vi "GetControlValue_DBL.vi"(8 "error in (no error)":errorcluster, 9 "Expected Data Type":dbl, 10 "Control Label":string, 11 "CtlLookup In":T1) -> (0 "error out":errorcluster, 2 "Value":dbl, 3 "CtlLookup Out":T1)   [LabVIEW 2018, in "CtlReferences.lvlib" / "CtlReferences.lvclass"]
doc: "This VI uses the GetControlByReference to get the specified control as a DBL"
uses:
  CtlReferences.lvclass
  TypeDefs/CtlLookup.ctl
  CtlReferences.lvclass/CtlReferences.ctl
  GetControlRef/GetControl_Control.vi
  GetControlRef/GetCtlRef_Base.vi
  GetCtlRef_Lookup.vi
  <vilib>/Utility/error.llb/Error Cluster From Error Code.vi
  Error_ToSpecificClass.vi
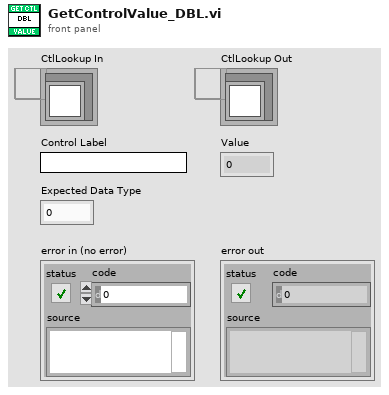
[diagram p1: front panel]
types:
  T1 = typedef "CtlReferences.lvlib/CtlReferences.lvclass/CtlLookup.ctl" = refnum<data-value>
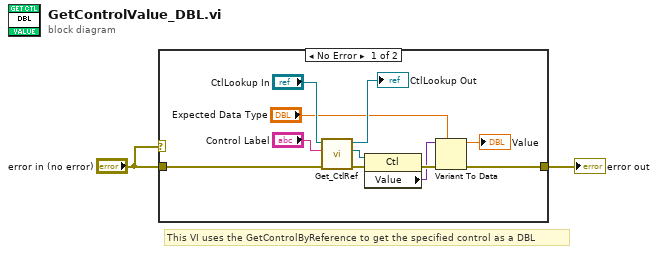
[diagram p0: block diagram]
diagram:
  # "This VI uses the GetControlByReference to get the specified control as a DBL"
  n1 = case shown="No Error" "error in (no error)" {
    tunnel: "error in (no error)" -> [w9 w14]
    tunnel: [w6 w14] -> w2
    frame No Error {
      n2 = call-poly "Get_CtlRef.vi"("error in (no error)"=w9, "Control Label"="Control Label", "CtlLookup In"="CtlLookup In") -> ("error out"=w12:errorcluster, "Reference Out"=w11:refnum<vi>, "CtlLookup Out"=→"CtlLookup Out":T1)  [unwired: 6 in]
      n3 = property class="Ctl"(reference=w11, error in=w12) -> (error out=w7:errorcluster, "Value"=w5:variant)  [unwired: 1 out]
      n4 = Variant To Data(error in=w7, type="Expected Data Type", Variant=w5) -> (data=→"Value":dbl, error out=w6:errorcluster)
    }
    frame Error {
    }
  }
  "error out" <- w2
